vi "SingleArrayToString.vi"(2 "SingleArrayOf6":sgl[](array[numeric])) -> (5 "1":string, 6 "2":string, 7 "3":string, 8 "6":string, 9 "4":string, 10 "5":string)   [LabVIEW 2016, in "M1M3SupportEUI_Views.lvlib"]
uses:
  M1M3SupportEUI_Views.lvlib
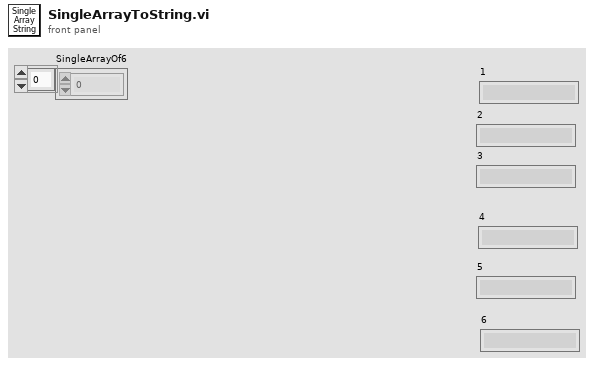
[diagram p1: front panel]
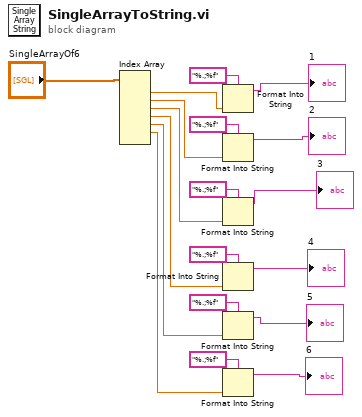
[diagram p0: block diagram]
diagram:
  n1 = Index Array(array="SingleArrayOf6") -> (element #1=w14:sgl, element #2=w15:sgl, element #3=w16:sgl, element #4=w17:sgl, element #5=w18:sgl, element #6=w19:sgl)  [unwired: 7 in, 1 out]
  n2 = Format Into String(format string="%.;%f", w14) -> (resulting string=→"1":string)  [unwired: 2 in, 1 out]
  n3 = Format Into String(format string="%.;%f", w15) -> (resulting string=→"2":string)  [unwired: 2 in, 1 out]
  n4 = Format Into String(format string="%.;%f", w16) -> (resulting string=→"3":string)  [unwired: 2 in, 1 out]
  n5 = Format Into String(format string="%.;%f", w17) -> (resulting string=→"4":string)  [unwired: 2 in, 1 out]
  n6 = Format Into String(format string="%.;%f", w18) -> (resulting string=→"5":string)  [unwired: 2 in, 1 out]
  n7 = Format Into String(format string="%.;%f", w19) -> (resulting string=→"6":string)  [unwired: 2 in, 1 out]
